vi "Edit Substeps Relay Output Common LTT Signals.vi"(8 "error in":errorcluster, 9 "Station No":i32, 10 "RelayOutputWrite":T1, 11 "Sequence Context In":refnum<k7>) -> (0 "error out":errorcluster, 2 "RelayOutputWrite Out":T1, 3 "Report Text":string)   [LabVIEW 2023, in "LTT_TeststandSteptypes.lvlib"]
uses:
  LTT_TeststandSteptypes.lvlib
  Control/Relay Output.ctl
  HardwareAbstractionLayer_LVOOP/Database/SQL Public VI/Control/DB Options.ctl
  <vilib>/addons/TestStand/_TSUtility.llb/TestStand - Start Modal Dialog (Sequence Context).vi
  <vilib>/addons/TestStand/_TSUtility.llb/TestStand - End Modal Dialog (Sequence Context).vi
  HardwareAbstractionLayer_LVOOP/Database/Database.lvclass
panel:
  in  "Close":bool
  in  "OK":bool
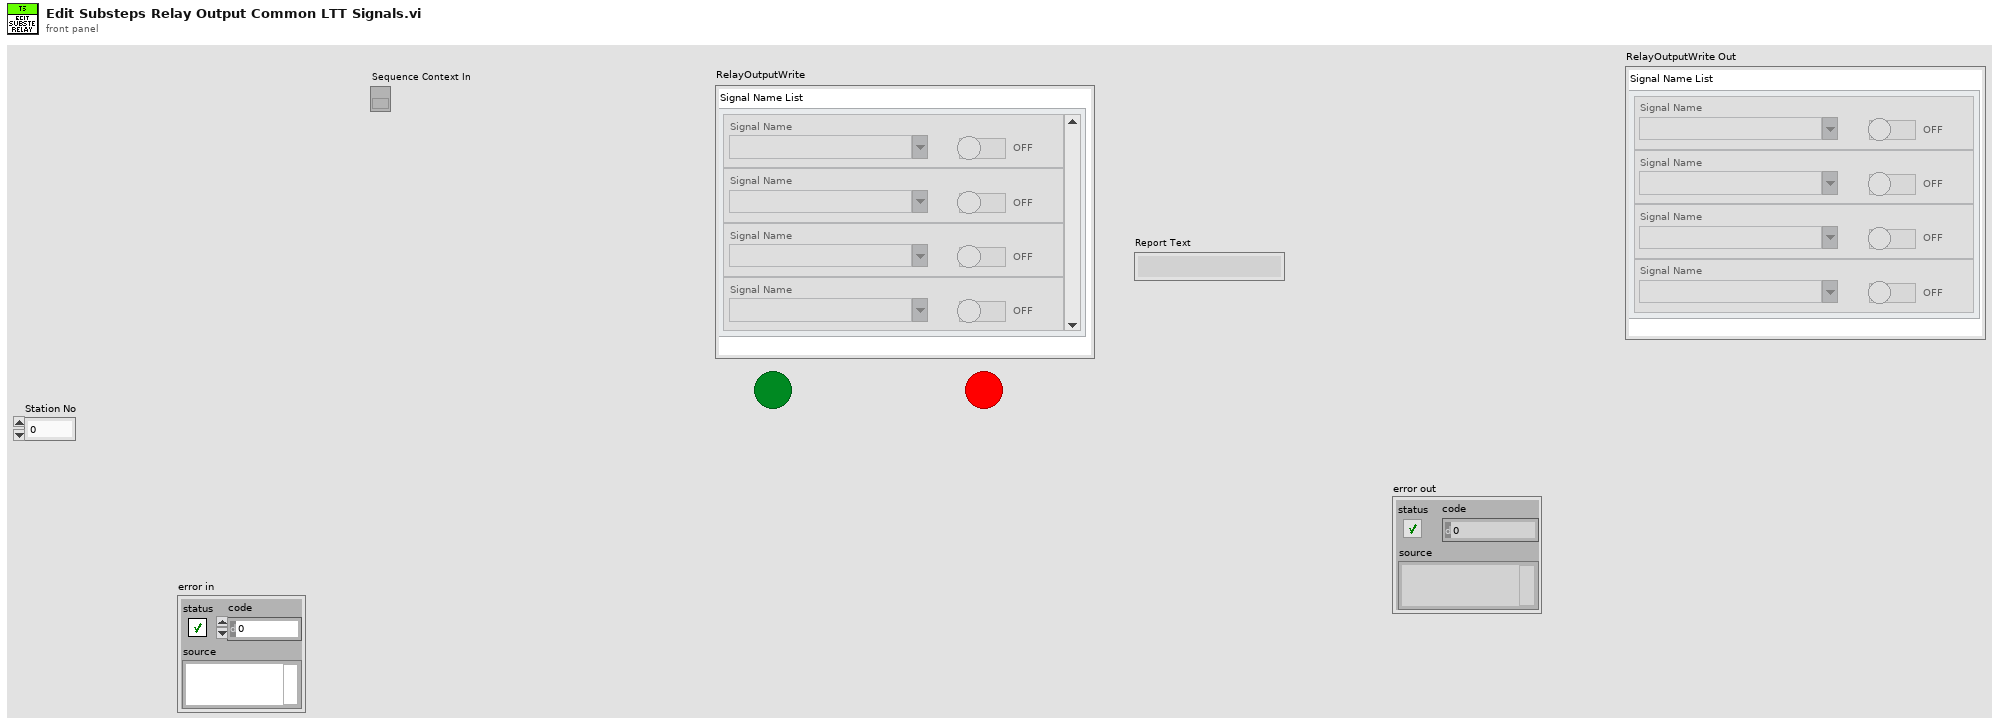
[diagram p1: front panel]
types:
  T1 = typedef "LTT_TeststandSteptypes.lvlib/Relay Output.ctl" = cluster{"Signal Name List":cluster{"Signal Name":string, "Enable Output":bool}[]}
  T2 = typedef "HardwareAbstractionLayer_LVOOP.lvlib/Database.lvclass/DB Options.ctl" = enum16{"Init", "Select Data", "Insert Data", "Update Data", "Delete Data", "Execute Query", "Create Schema", "Create Table", "List Tables", "List Columns", "Close"}
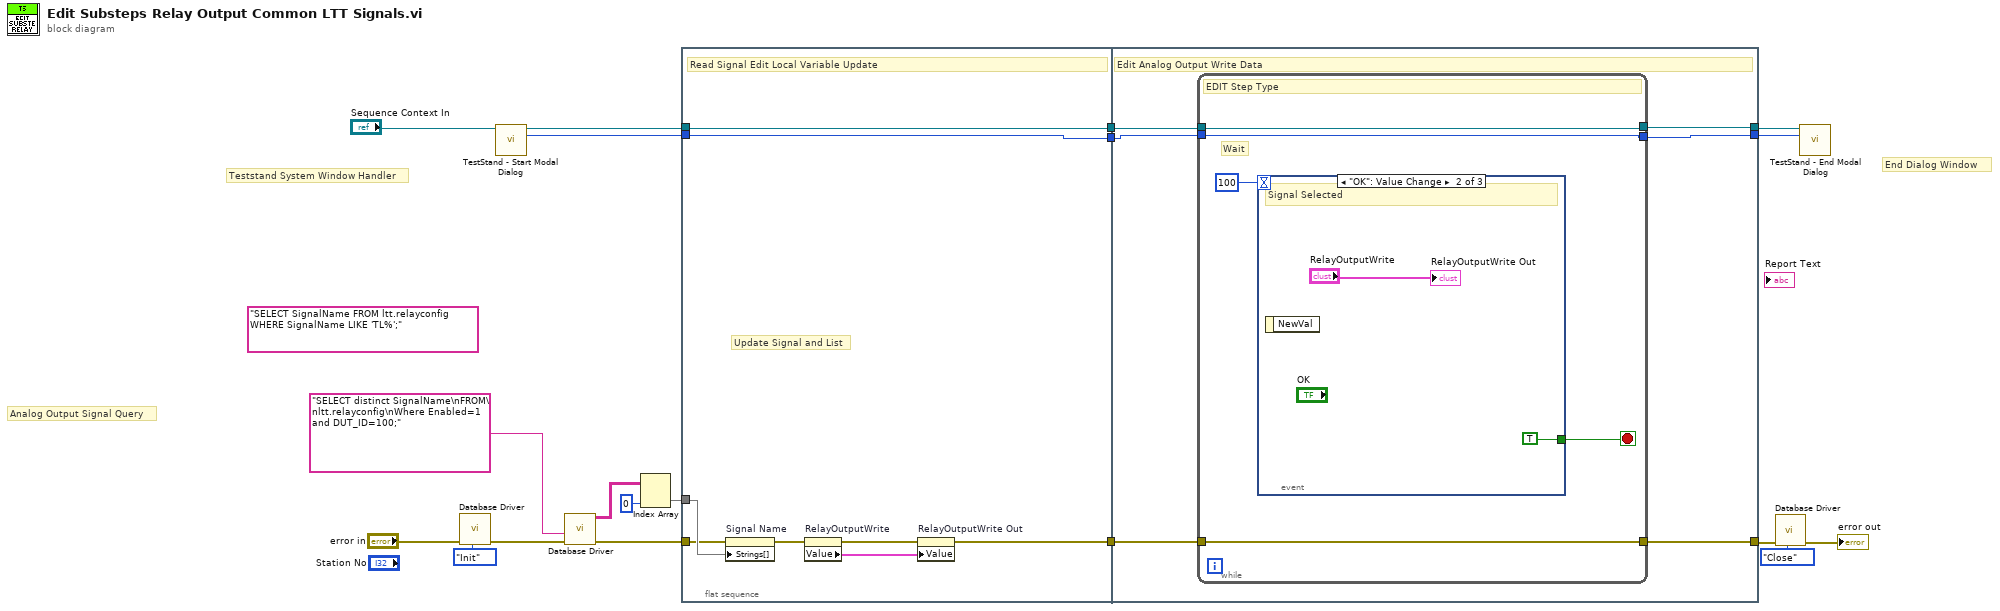
[diagram p0: block diagram]
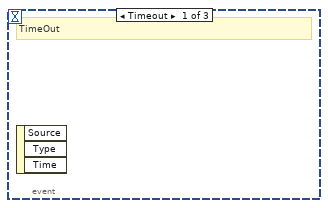
[diagram p2: hidden frame]
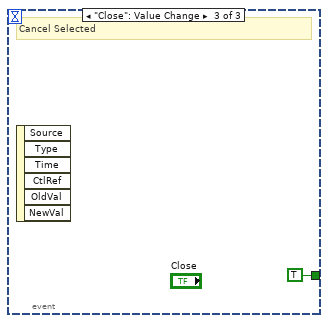
[diagram p3: hidden frame]
diagram:
  (unwired) "SELECT SignalName FROM ltt.relayconfig WHERE SignalName LIKE 'TL%';" ("SQL query")
  # "Teststand System Window Handler"
  # "End Dialog Window"
  # "Analog Output Signal Query"
  n1 = call "Database Driver.vi"("Options"=DB_Options."Init", "error in"="error in") -> ("error out"=w6:errorcluster)  [unwired: 6 in, 3 out]
  n2 = call-poly <vilib>:"TestStand - Start Modal Dialog.vi"("Sequence Context In"="Sequence Context In") -> ("Sequence Context Out"=w15:refnum<k7>, "Modal ID"=w14:i32)  [unwired: 10 in, 3 out]
  n3 = call "Database Driver.vi"("error in"=w6, "SQL query"="SELECT distinct SignalName\nFROM\nltt.relayconfig\nWhere Enabled=1 and DUT_ID=100;") -> ("error out"=w11:errorcluster, "data"=w10:string[][])  [unwired: 6 in, 2 out]
  n4 = Index Array(array=w10, index (col)=0 ("disabled index (col)")) -> (element=w9:string[])  [unwired: 1 in]
  n5 = flat-sequence {
    tunnel: w11 -> [w24]
    tunnel: [w20] -> w19
    tunnel: w15 -> [w27]
    tunnel: [w27] -> w17
    tunnel: w9 -> [w25]
    tunnel: w14 -> [w26]
    tunnel: [w26] -> w13
    tunnel: w19 -> [w33]
    tunnel: [w32] -> w18
    tunnel: w17 -> [w31]
    tunnel: [w30] -> w16
    tunnel: w13 -> [w29]
    tunnel: [w28] -> w12
    frame #0 {
      # "Update Signal and List"
      # "Read Signal Edit Local Variable Update"
      n6 = property on="Signal Name" class="CmbBox"(error in=w24, "Strings[]"=w25) -> (error out=w22:errorcluster)  [unwired: 1 in, 1 out]
      n7 = property on="RelayOutputWrite" class="Clust (strict)"(error in=w22) -> (error out=w21:errorcluster, "Value"=w23:T1)  [unwired: 1 in, 1 out]
      n8 = property on="RelayOutputWrite Out" class="Clust (strict)"(error in=w21, "Value"=w23) -> (error out=w20:errorcluster)  [unwired: 1 in, 1 out]
    }
    frame #1 {
      # "Edit Analog Output Write Data"
      n9 = while {
        tunnel: w33 -> [w38]
        tunnel: [w38] -> w32
        tunnel: w31 -> [w37]
        tunnel: [w37] -> w30
        tunnel: w29 -> [w34]
        tunnel: [w34] -> w28
        stop <- w35 stop-if-true
        # "Wait"
        # "EDIT Step Type"
        n10 = event shown="[1] \"OK\": Value Change" {
          selector: _ -> [_ _ _]
          dyn-events: _ -> [_ _ _]
          timeout: 100 -> [_ _ _]
          tunnel: [_ TRUE ("Stop") TRUE ("Stop")] -> w35
          event Timeout {
            # "TimeOut"
            n11 = event-data() -> ()  [unwired: 1 in, 3 out]
          }
          event "OK": Value Change {
            # "Signal Selected"
            n12 = event-data() -> ()  [unwired: 1 in, 1 out]
            "RelayOutputWrite Out" <- "RelayOutputWrite"
          }
          event "Close": Value Change {
            # "Cancel Selected"
            n13 = event-data() -> ()  [unwired: 1 in, 6 out]
          }
        }
      }
    }
  }
  n14 = call "Database Driver.vi"("Options"=DB_Options."Close", "error in"=w18) -> ("error out"=→"error out":errorcluster)  [unwired: 6 in, 3 out]
  n15 = call-poly <vilib>:"TestStand - End Modal Dialog.vi"("Sequence Context In"=w16, "Modal ID"=w12) -> ()  [unwired: 13 in, 1 out]
